vi "FormatJoystick.vi"(8 "error in (no error)":errorcluster, 11 "Refnum in":refnum<k1>) -> (0 "Speed Cap":dbl, 1 "FZ":dbl(slide) scale=-1.0..1.0, 2 "FXY":cluster{"X":dbl, "Y":dbl}[](graph), 3 "Axes":cluster{"X":dbl, "Y":dbl, "Z":dbl})   [LabVIEW 2014]
uses:
  <vilib>/Utility/inputDevices.llb/joystickAcquire.vi
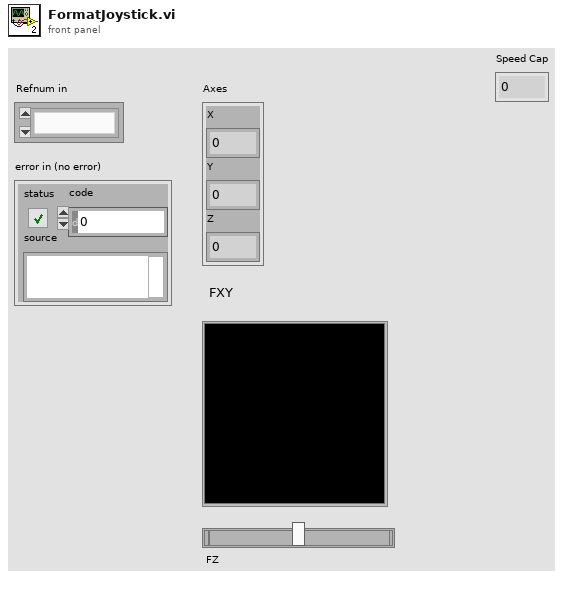
[diagram p1: front panel]
types:
  T1 = cluster{"X axis":i32, "Y axis":i32, "Z axis":i32, "X axis rotation":i32, "Y axis rotation":i32, "Z axis rotation":i32, "U axis":i32, "V axis":i32}
  T2 = cluster{"X axis":dbl, "Y axis":dbl, "Z axis":dbl, "X axis rotation":dbl, "Y axis rotation":dbl, "Z axis rotation":dbl, "U axis":dbl, "V axis":dbl}
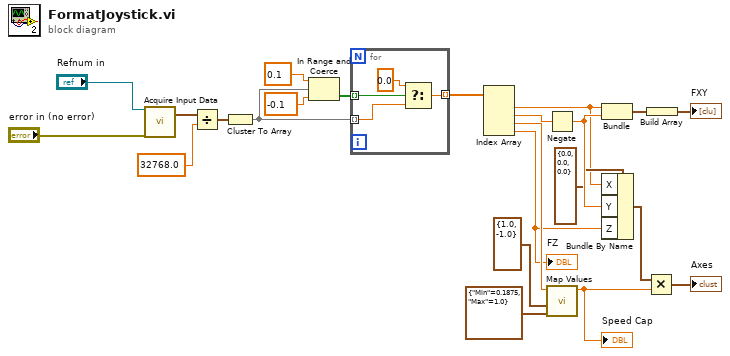
[diagram p0: block diagram]
diagram:
  n1 = call-poly <vilib>:"Acquire Input Data.vi"("device ID"="Refnum in", "error in (no error)"="error in (no error)") -> ("axis info"=w19:T1)  [unwired: 13 in, 4 out]
  n2 = Divide(x=w19, y=32768.0) -> (x/y=w10:T2)
  n3 = Cluster To Array(cluster=w10) -> (array=w6:dbl[])
  n4 = In Range and Coerce(upper limit=0.1, x=w6, lower limit=-0.1) -> (In Range?=w7:bool[])  [unwired: 1 out]
  n5 = for {
    tunnel: w7 -> [w27] mode=indexing
    tunnel: w6 -> [w25] mode=indexing
    tunnel: [w24] -> w3 mode=indexing
    n6 = Select(t=0.0, s=w27, f=w25) -> (s? t:f=w24:dbl)
  }
  n7 = Index Array(array=w3) -> (element #1=w5:dbl, element #2=w4:dbl, element #3=w2:dbl, element #4=w1:dbl)  [unwired: 4 in]
  "FZ" <- w1
  n8 = Negate(x=w4) -> (-x=w21:dbl)
  n9 = call "Map Values.vi"("Output"=cluster{"Min":dbl, "Max":dbl} {"Min"=0.1875, "Max"=1.0}, "Input"=cluster{"Min":dbl, "Max":dbl} {"Min"=1.0, "Max"=-1.0}, "Value"=w2) -> ("Mapped Value"=w12:dbl)  [unwired: 8 in]
  "Speed Cap" <- w12
  n10 = Bundle("X axis"=w5, w21) -> (w23:cluster{"X axis":dbl, dbl})  [unwired: 1 in]
  n11 = Bundle By Name(cluster=cluster{"X":dbl, "Y":dbl, "Z":dbl} {"X"=0.0, "Y"=0.0, "Z"=0.0} ("Axes"), "X"=w5, "Y"=w21, "Z"=w1) -> (w13:cluster{"X":dbl, "Y":dbl, "Z":dbl})
  n12 = Multiply(x=w13, y=w12) -> (x*y=→"Axes":cluster{"X":dbl, "Y":dbl, "Z":dbl})
  n13 = Build Array(w23) -> (→"FXY":cluster{"X axis":dbl, dbl}[])
